vi "Test 1 First Step Col.vi"(8 "error in (no error)":errorcluster, 11 "Test Case In":refnum<class "Tests.lvclass">) -> (0 "error out":errorcluster, 3 "Test Case Out":refnum<class "Tests.lvclass">)   [LabVIEW 2021, in "Tests.lvclass"]
uses:
  Tests.lvclass
  Tests.lvclass/Tests.ctl
  4993e8ee-a06a-463a-9684-69129f64d5ce.vi
  Proto/Proto.lvclass
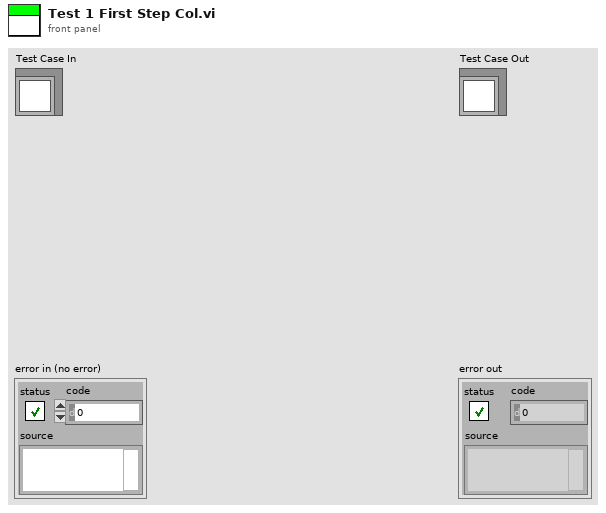
[diagram p1: front panel]
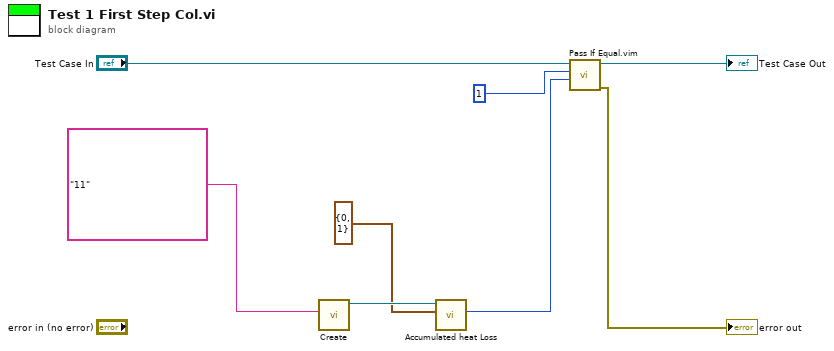
[diagram p0: block diagram]
diagram:
  n1 = call "Create.vi"("Input"="11") -> ("Proto"=w5:refnum<class "Proto.lvclass">)  [unwired: 10 in]
  n2 = call "Accumulated heat Loss.vi"("Coord"=cluster{"Row":i32, "Col":i32} {"Row"=0, "Col"=1}, "Proto in"=w5) -> ("Min Heat"=w2:i32)  [unwired: 8 in, 1 out]
  n3 = call "Pass If Equal.vim"("Actual"=w2, "Expected"=1 ("Heat"), "LUnit Test Case In"="Test Case In") -> ("error out"=→"error out":errorcluster, "LUnit Test Case Out"=→"Test Case Out":refnum<class "Tests.lvclass">)  [unwired: 7 in]
